vi "SCOnly.vi"() -> ()   [LabVIEW 2014]
uses:
  <vilib>/Instr/_visa.llb/VISA Configure Serial Port (Instr).vi
panel:
  in  "stop":bool
  in  "Abort SC":bool
  out "Si Abort Readout":string
  out "TL Abort readout":string
  in  "Si Test Steps":dbl format="%#_13g"
  out "Si Test String":string
  out "Si Test Readout":string
  in  "Si Test":bool=TRUE
  in  "TL Test Steps":dbl format="%#_13g"
  out "Tl Test String":string
  out "Tl Test Readout":string
  in  "TL Test":bool=TRUE
  in  "Si":T1(radio)=enum."Radio Selection 1"
  out "Si in Position? SC":bool=TRUE
  out "TL in Position? SC":bool=TRUE
  in  "Normal/Overide":bool=TRUE
  in  "TL":T2(radio)=enum."Radio Selection 1"
  out "Si Output":string
  out "Si Input":string
  out "TL Output":string
  out "TL Input":string
  in  "Pos5 Enable":bool=TRUE
  in  "Pos4 Enable":bool=TRUE
  in  "Pos3 Enable":bool=TRUE
  in  "Pos2 Enable":bool=TRUE
  in  "Pos1 Enable":bool=TRUE
  out "Si Position Readout":string
  out "TL Position Readout":string
  out "TL Position":i32
  out "TL Bar":i32(slide) scale=0.0..429000.0
  out "Si Position":i32
  out "Si Bar":i32(slide) scale=0.0..49001.0
  in  "SC On/Off":bool=TRUE
  in  "Si Speed Value":i32=2000
  in  "Si MID Value":i32=26000
  in  "Si IN Value":i32=49000
  in  "TL Speed Value":i32=4000
  in  "Pos5 Value":i32=429000
  in  "Pos4 Value":i32=339000
  in  "Pos3 Value":i32=249000
  in  "Pos2 Value":i32=163000
  in  "Pos1 Value":i32=71000
  out "Si \nSpeed":i32 min=0 format="%#.10f"
  out "Si MID":i32 min=0 format="%#.10f"
  out "Si IN":i32 min=0 format="%#.10f"
  out "TL \nSpeed":i32 min=0 format="%#.10f"
  out "Position5":i32 min=0 format="%#.10f"
  out "Position4":i32 min=0 format="%#.10f"
  out "Position3":i32 min=0 format="%#.10f"
  out "Position2":i32 min=0 format="%#.10f"
  out "Position1":i32 min=0 format="%#.10f"
  in  "TL/Si, Comm 29, C":refnum<visa-resource-name>="COM29"
  # "Faraday Cup"
  # "Si Home"
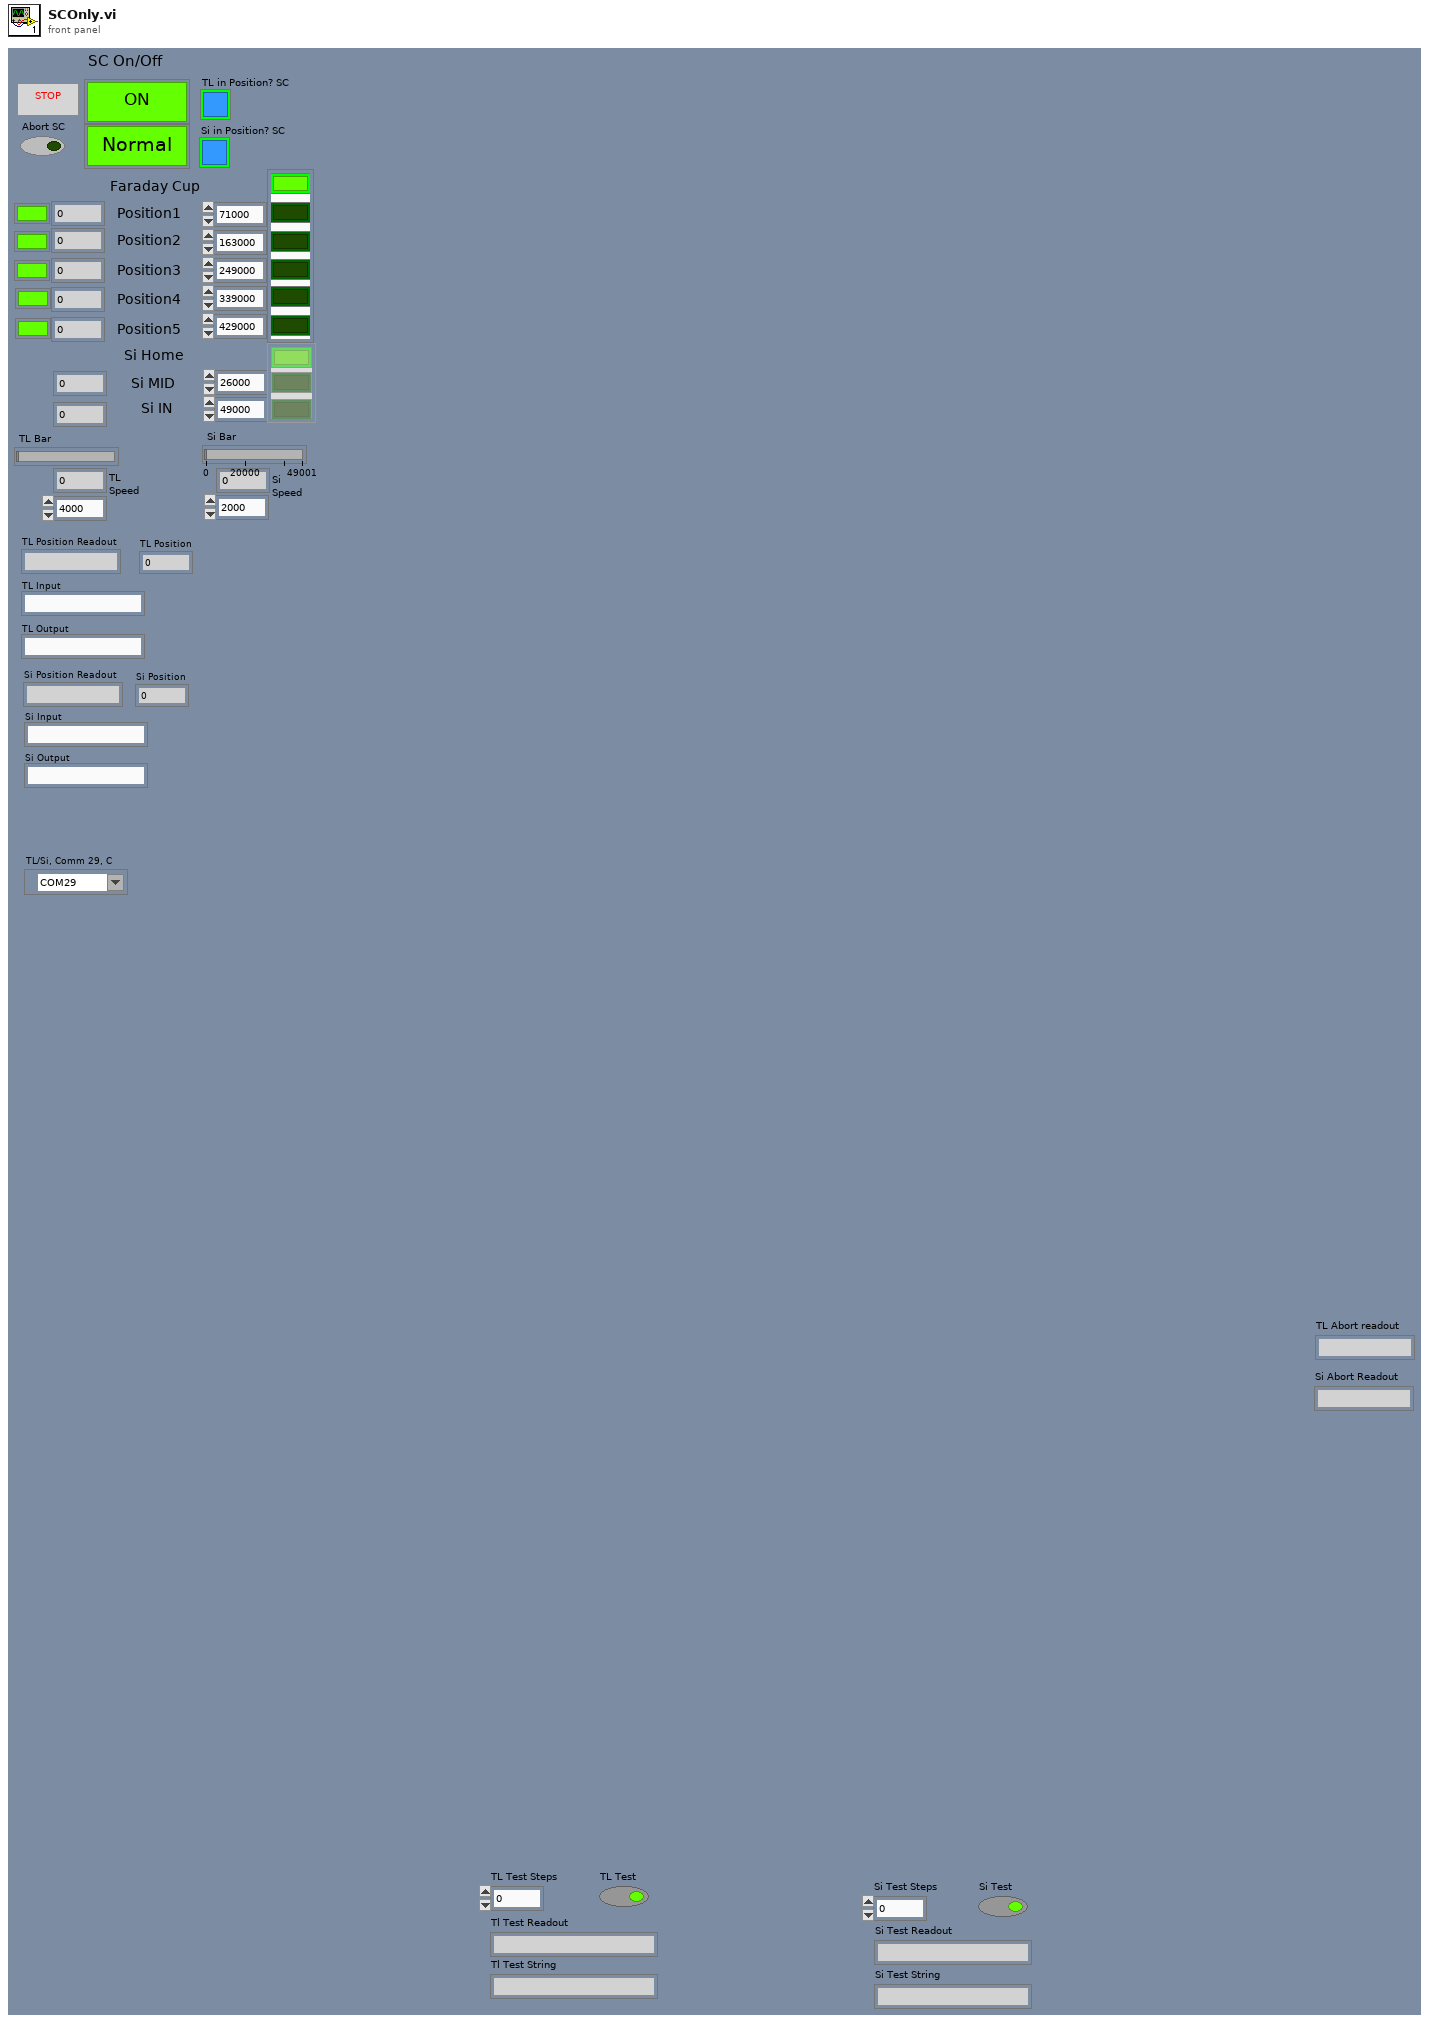
[diagram p1: front panel]
types:
  T1 = enum32{"No Selection", "Radio Selection 1", "Radio Selection 2", "Radio Selection 3"}
  T2 = enum32{"No Selection", "Radio Selection 1", "Radio Selection 2", "Radio Selection 3", "Radio Selection 4", "Radio Selection 5", "Radio Selection 6"}
  T3 = enum8{"Enabled", "Disabled", "Disabled and Grayed Out"}
  T4 = cluster{"read buffer":string, "Numeric":i32, "read buffer":string, "Numeric":i32, bool}
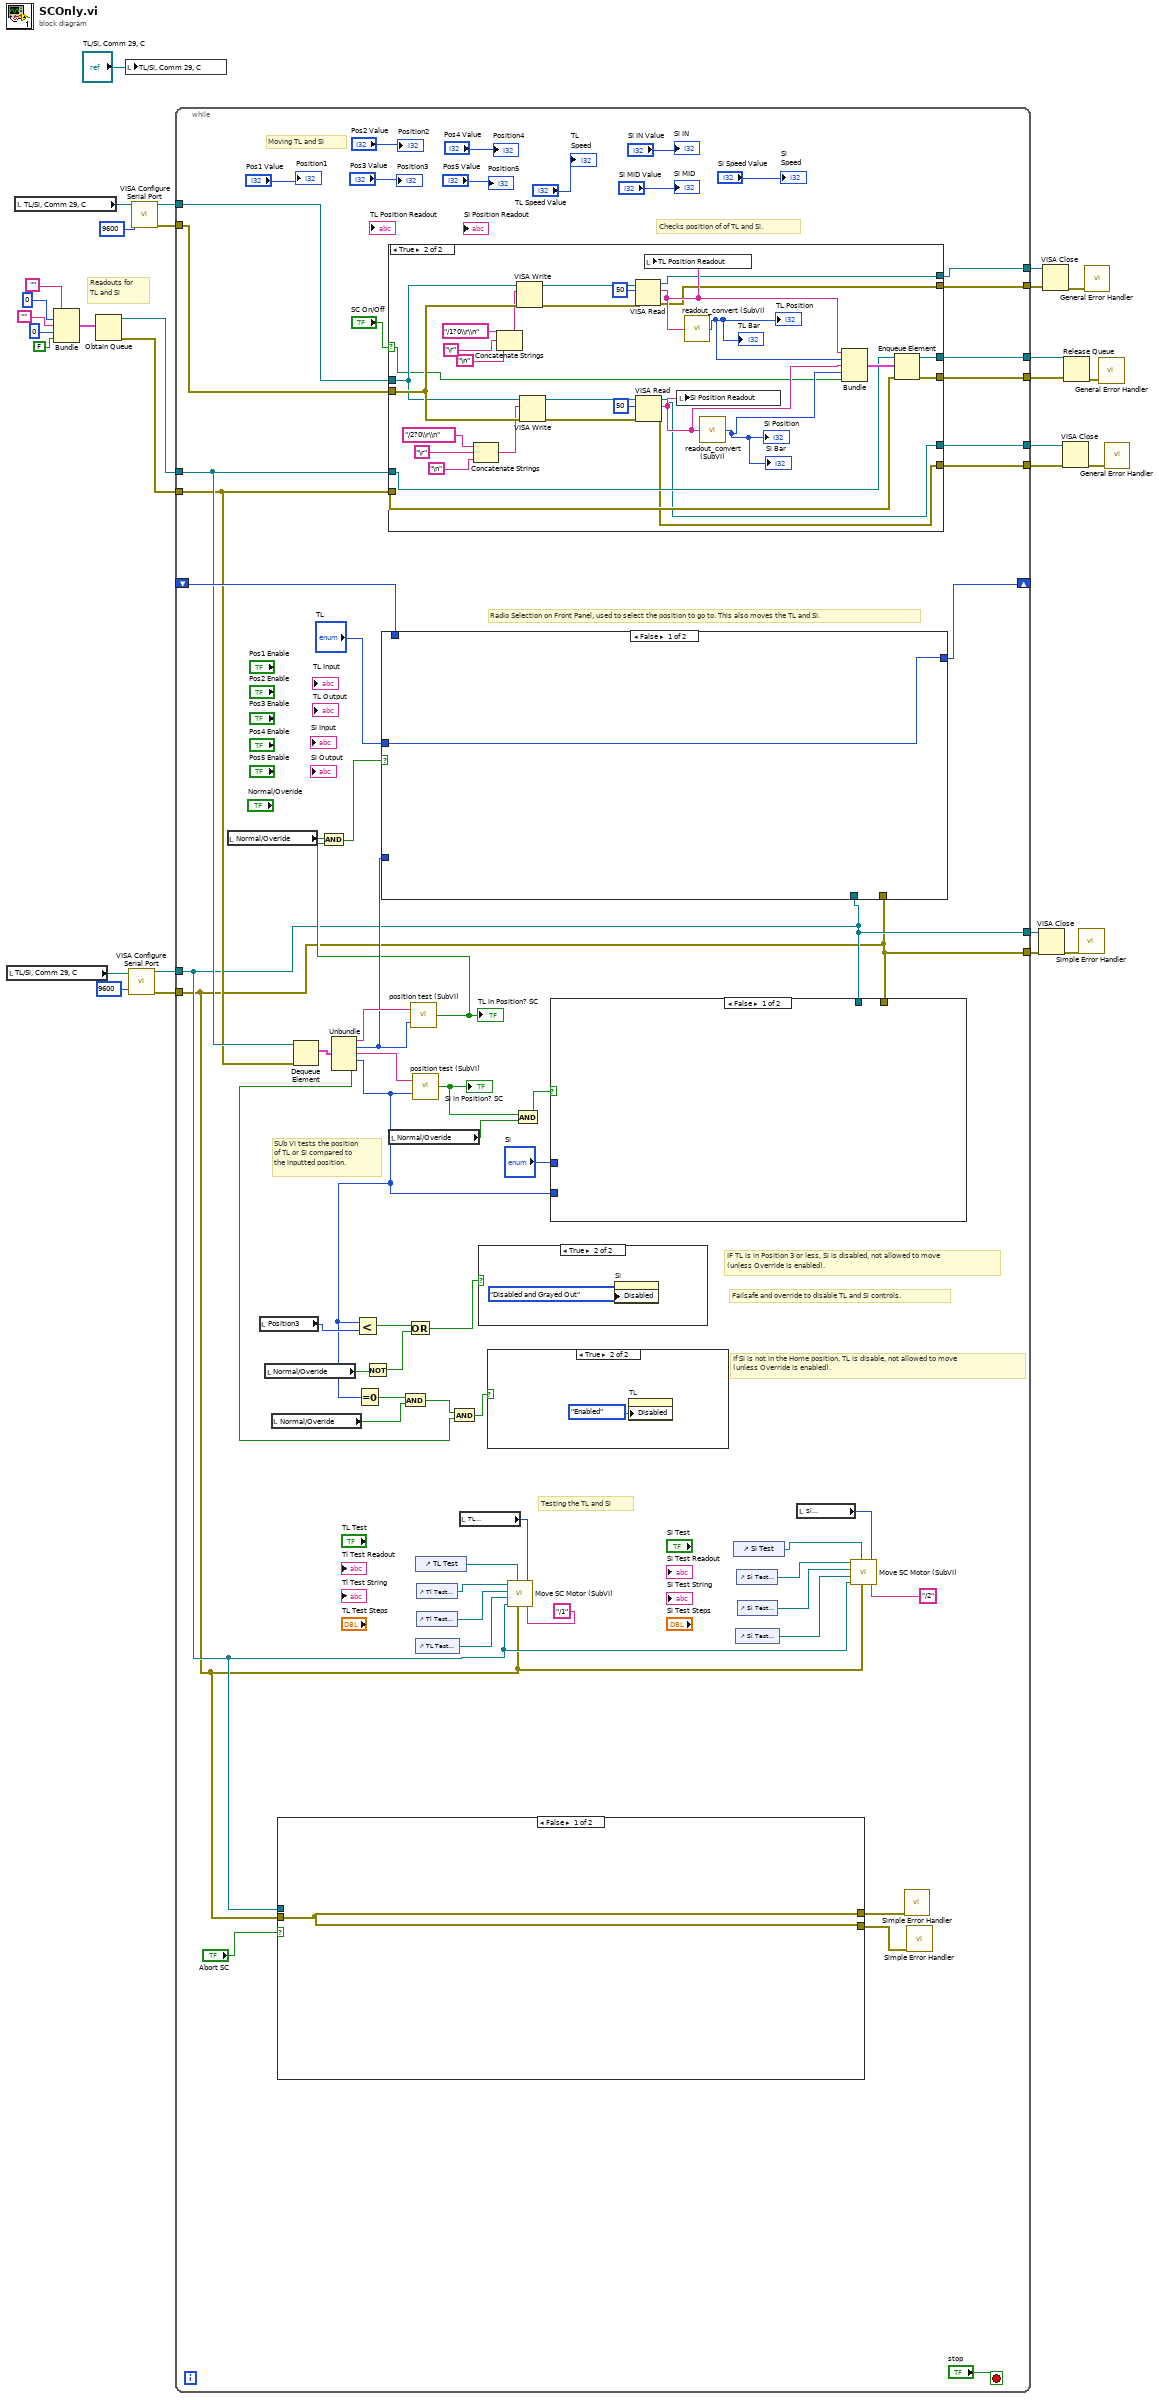
[diagram p0: block diagram]
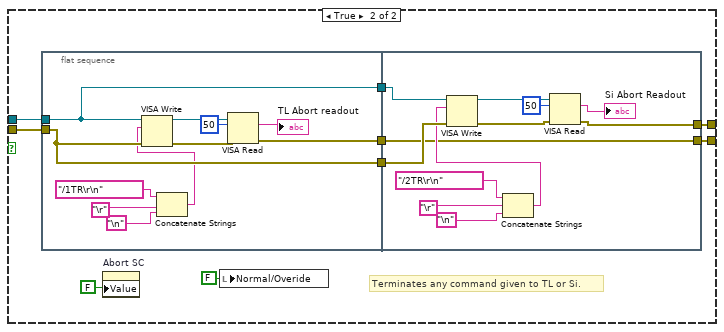
[diagram p2: hidden frame]
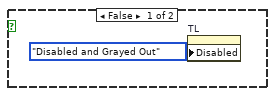
[diagram p3: hidden frame]
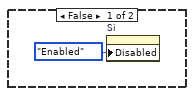
[diagram p4: hidden frame]
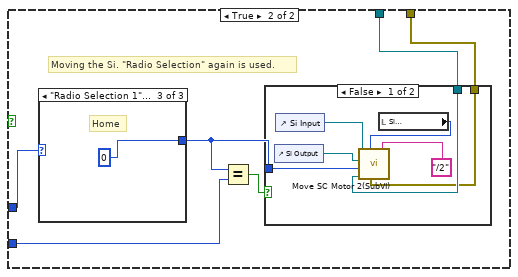
[diagram p5: hidden frame]
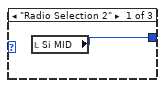
[diagram p7: hidden frame]
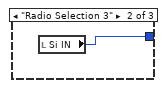
[diagram p8: hidden frame]
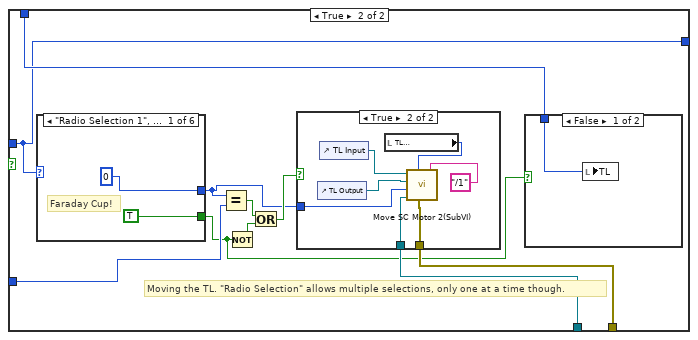
[diagram p9: hidden frame]
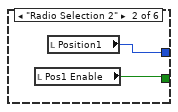
[diagram p12: hidden frame]
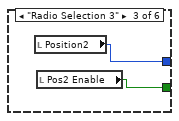
[diagram p13: hidden frame]
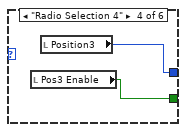
[diagram p14: hidden frame]
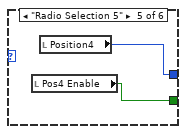
[diagram p15: hidden frame]
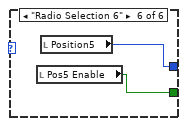
[diagram p16: hidden frame]
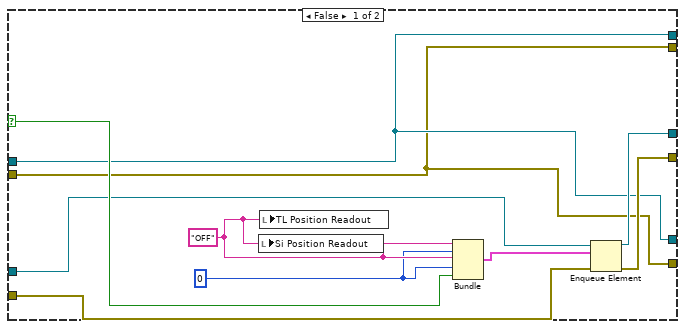
[diagram p17: hidden frame]
diagram:
  # "Readouts for \nTL and Si"
  n1 = local read "TL/Si, Comm 29, C"() -> (w11:refnum<visa-resource-name>)
  n2 = local read "TL/Si, Comm 29, C"() -> (w28:refnum<visa-resource-name>)
  n3 = Bundle("", 0, "", 0, FALSE) -> (w20:cluster{string, i32, string, i32, bool})  [unwired: 1 in]
  n4 = Obtain Queue(element data type=w20) -> (queue out=w19:refnum<queue>, error out=w18:errorcluster)  [unwired: 4 in, 1 out]
  n5 = local write "TL/Si, Comm 29, C"("TL/Si, Comm 29, C") -> ()
  n6 = call-poly "VISA Configure Serial Port"("VISA resource name"=w11, "baud rate (9600)"=u32 9600) -> ("VISA resource name out"=w10:refnum<visa-resource-name>, "error out"=w9:errorcluster)  [unwired: 12 in]
  n7 = call-poly "VISA Configure Serial Port"("VISA resource name"=w28, "baud rate (9600)"=u32 9600) -> ("VISA resource name out"=w27:refnum<visa-resource-name>, "error out"=w26:errorcluster)  [unwired: 12 in]
  n8 = while {
    tunnel: w27 -> [w81]
    tunnel: w26 -> [w82]
    tunnel: w19 -> [w70]
    tunnel: w18 -> [w69]
    tunnel: [w80] -> w15
    tunnel: [w79] -> w14
    tunnel: [w78] -> w13
    tunnel: [w77] -> w12
    shift-right: [w72] -> _
    shift-left: _ -> [w73]
    tunnel: w10 -> [w34]
    tunnel: w9 -> [w33]
    tunnel: [w34] -> w7
    tunnel: [w33] -> w6
    tunnel: [w31] -> w4
    tunnel: [w30] -> w3
    stop <- "stop" stop-if-true
    # "Testing the TL and Si"
    # "If Si is not in the Home position, TL is disable, not allowed to move\n(unless Override is enabled)."
    # "Failsafe and override to disable TL and Si controls."
    # "IF TL is in Position 3 or less, Si is disabled, not allowed to move\n(unless Override is enabled)."
    # "SUb Vi tests the position\nof TL or Si compared to\nthe inputted position."
    # "Radio Selection on Front Panel, used to select the position to go to. This also moves the TL and Si."
    # "Checks position of of TL and Si."
    # "Moving TL and Si"
    n9 = local read "Normal/Overide"() -> (w76:bool)
    n10 = local read "Position3"() -> (w60:i32)
    n11 = local read "Normal/Overide"() -> (w58:bool)
    n12 = local read "Normal/Overide"() -> (w54:bool)
    n13 = case shown="False" "Abort SC" {
      tunnel: w34 -> [_ w102]
      tunnel: w33 -> [w93 w100]
      tunnel: [w93 w97] -> w36
      tunnel: [w93 w96] -> w37
      frame False {
      }
      frame True {
        # "Terminates any command given to TL or Si."
        n14 = flat-sequence {
          tunnel: w102 -> [w112]
          tunnel: [w112] -> w101
          tunnel: w100 -> [w110]
          tunnel: [w110] -> w99
          tunnel: [w103] -> w98
          tunnel: w101 -> [w125]
          tunnel: w99 -> [w123]
          tunnel: w98 -> [w115]
          tunnel: [w115] -> w97
          tunnel: [w114] -> w96
          frame #0 {
            n15 = Concatenate Strings("/1TR\r\n", "\r", "\n") -> (w105:string)
            n16 = VISA Write(VISA resource name=w112, write buffer=w105, error in (no error)=w110) -> (VISA resource name out=w113:refnum<visa-resource-name>, error out=w111:errorcluster)  [unwired: 1 out]
            n17 = VISA Read(VISA resource name=w113, byte count=u32 50, error in (no error)=w111) -> (read buffer=→"TL Abort readout":string, error out=w103:errorcluster)  [unwired: 2 out]
          }
          frame #1 {
            n18 = Concatenate Strings("/2TR\r\n", "\r", "\n") -> (w117:string)
            n19 = VISA Write(VISA resource name=w125, write buffer=w117, error in (no error)=w123) -> (VISA resource name out=w124:refnum<visa-resource-name>, error out=w122:errorcluster)  [unwired: 1 out]
            n20 = VISA Read(VISA resource name=w124, byte count=u32 50, error in (no error)=w122) -> (read buffer=→"Si Abort Readout":string, error out=w114:errorcluster)  [unwired: 2 out]
          }
        }
        n21 = property on="Abort SC" class="Bool (strict)"("Value"=FALSE ("Abort SC")) -> ()  [unwired: 2 in, 2 out]
        n22 = local write "Normal/Overide"(FALSE ("Normal/Overide")) -> ()
      }
    }
    n23 = Dequeue Element(queue=w70, error in (no error)=w69) -> (element=w71:cluster{string, i32, string, i32, bool})  [unwired: 1 in, 3 out]
    n24 = Unbundle(w71) -> (w68:string, w66:i32, w67:string, w56:i32, w52:bool)
    n25 = Less?(x=w56, y=w60) -> (x < y?=w59:bool)
    n26 = Equal To 0?(x=w56) -> (x = 0?=w55:bool)
    n27 = Not(x=w58) -> (.not. x?=w57:bool)
    n28 = case shown="True" "SC On/Off" {
      selector: "SC On/Off" -> [w184 w193]
      tunnel: w81 -> [w178 w212]
      tunnel: w82 -> [w177 w216]
      tunnel: w70 -> [w182 w201]
      tunnel: w69 -> [w181 w200]
      tunnel: [w180 w199] -> w78
      tunnel: [w179 w198] -> w77
      tunnel: [w178 w196] -> w80
      tunnel: [w177 w197] -> w79
      tunnel: [w178 w195] -> w31
      tunnel: [w177 w194] -> w30
      frame False {
        w185 = 0
        w186 = "OFF"
        n29 = local write "Si Position Readout"(w186) -> ()
        n30 = local write "TL Position Readout"(w186) -> ()
        n31 = Bundle(w186, w185, w186, w185, w184) -> (w183:cluster{string, i32, string, i32, bool})  [unwired: 1 in]
        n32 = Enqueue Element(queue=w182, element=w183, error in (no error)=w181) -> (queue out=w180:refnum<queue>, error out=w179:errorcluster)  [unwired: 1 in, 1 out]
      }
      frame True {
        n33 = Concatenate Strings("/2?0\\r\\n", "\r", "\n") -> (w205:string)
        n34 = Concatenate Strings("/1?0\\r\\n", "\r", "\n") -> (w211:string)
        n35 = VISA Write(VISA resource name=w212, write buffer=w211, error in (no error)=w216) -> (VISA resource name out=w192:refnum<visa-resource-name>, error out=w191:errorcluster)  [unwired: 1 out]
        n36 = VISA Write(VISA resource name=w212, write buffer=w205, error in (no error)=w216) -> (VISA resource name out=w189:refnum<visa-resource-name>, error out=w188:errorcluster)  [unwired: 1 out]
        n37 = VISA Read(VISA resource name=w192, byte count=u32 50, error in (no error)=w191) -> (VISA resource name out=w196:refnum<visa-resource-name>, read buffer=w210:string, error out=w197:errorcluster)  [unwired: 1 out]
        n38 = VISA Read(VISA resource name=w189, byte count=u32 50, error in (no error)=w188) -> (VISA resource name out=w195:refnum<visa-resource-name>, read buffer=w204:string, error out=w194:errorcluster)  [unwired: 1 out]
        n39 = local write "TL Position Readout"(w210) -> ()
        n40 = local write "Si Position Readout"(w204) -> ()
        n41 = call "readout_convert (SubVI).vi"("read buffer"=w210) -> ("Numeric"=w209:i32)
        "TL Position" <- w209
        "TL Bar" <- w209
        n42 = call "readout_convert (SubVI).vi"("read buffer"=w204) -> ("Numeric"=w203:i32)
        "Si Position" <- w203
        "Si Bar" <- w203
        n43 = Bundle("read buffer"=w210, "Numeric"=w209, "read buffer"=w204, "Numeric"=w203, w193) -> (w202:T4)  [unwired: 1 in]
        n44 = Enqueue Element(queue=w201, element=w202, error in (no error)=w200) -> (queue out=w199:refnum<queue>, error out=w198:errorcluster)  [unwired: 1 in, 1 out]
      }
    }
    n45 = local read "Normal/Overide"() -> (w61:bool)
    n46 = And(x=w55, y=w54) -> (x .and. y?=w53:bool)
    n47 = Or(x=w59, y=w57) -> (x .or. y?=w51:bool)
    n48 = call "position test (SubVI).vi"("Numeric"=w66, "String"=w68) -> ("Boolean"=w65:bool)
    "TL in Position? SC" <- w65
    n49 = And(x=w76, y=w65) -> (x .and. y?=w75:bool)
    n50 = case shown="False" w75 {
      tunnel: "TL" -> [w146 w152]
      tunnel: w73 -> [_ w153]
      tunnel: [w146 w152] -> w72
      tunnel: w66 -> [_ w151]
      tunnel: w34 -> [_ w149]
      tunnel: w33 -> [_ w148]
      frame False {
      }
      frame True {
        # "Moving the TL. \"Radio Selection\" allows multiple selections, only one at a time though."
        n51 = case shown="\"Radio Selection 1\", Default" w152 {
          tunnel: [0 w168 w170 w172 w174 w176] -> w150
          tunnel: [TRUE w167 w169 w171 w173 w175] -> w147
          frame "Radio Selection 1", Default {
            # "Faraday Cup!"
          }
          frame "Radio Selection 2" {
            n52 = local read "Pos1 Enable"() -> (w167:bool)
            n53 = local read "Position1"() -> (w168:i32)
          }
          frame "Radio Selection 3" {
            n54 = local read "Position2"() -> (w170:i32)
            n55 = local read "Pos2 Enable"() -> (w169:bool)
          }
          frame "Radio Selection 4" {
            n56 = local read "Pos3 Enable"() -> (w171:bool)
            n57 = local read "Position3"() -> (w172:i32)
          }
          frame "Radio Selection 5" {
            n58 = local read "Pos4 Enable"() -> (w173:bool)
            n59 = local read "Position4"() -> (w174:i32)
          }
          frame "Radio Selection 6" {
            n60 = local read "Pos5 Enable"() -> (w175:bool)
            n61 = local read "Position5"() -> (w176:i32)
          }
        }
        n62 = Equal?(x=w150, y=w151) -> (x = y?=w154:bool)
        n63 = Not(x=w147) -> (.not. x?=w155:bool)
        n64 = Or(x=w154, y=w155) -> (x .or. y?=w156:bool)
        n65 = case shown="True" w156 {
          tunnel: w150 -> [_ w160]
          tunnel: w149 -> [_ w159]
          tunnel: w148 -> [_ w158]
          frame False {
          }
          frame True {
            n66 = control-ref of="TL Output"() -> (w163:refnum<vi>)
            n67 = control-ref of="TL Input"() -> (w164:refnum<vi>)
            n68 = local read "TL \nSpeed"() -> (w162:i32)
            n69 = call "Move SC Motor 2(SubVI).vi"("String"="/1", "error out"=w158, "Speed"=w162, "VISA resource name out"=w159, "Position"=w160, "Output"=w163, "Input"=w164) -> ()
          }
        }
        n70 = case shown="False" w147 {
          tunnel: w153 -> [w157 _]
          frame False {
            n71 = local write "TL"(w157) -> ()
          }
          frame True {
          }
        }
      }
    }
    n72 = call "position test (SubVI).vi"("Numeric"=w56, "String"=w67) -> ("Boolean"=w62:bool)
    "Si in Position? SC" <- w62
    n73 = control-ref of="TL Test Steps"() -> (w45:refnum<vi>)
    n74 = control-ref of="TL Test"() -> (w48:refnum<vi>)
    n75 = control-ref of="Tl Test Readout"() -> (w47:refnum<vi>)
    n76 = control-ref of="Tl Test String"() -> (w46:refnum<vi>)
    n77 = And(x=w53, y=w52) -> (x .and. y?=w50:bool)
    n78 = local read "TL \nSpeed"() -> (w49:i32)
    n79 = case shown="True" w51 {
      frame False {
        n80 = property on="Si" class="RadioBtnsControl (strict)"("Disabled"=T3."Enabled") -> ()  [unwired: 2 in, 2 out]
      }
      frame True {
        n81 = property on="Si" class="RadioBtnsControl (strict)"("Disabled"=T3."Disabled and Grayed Out") -> ()  [unwired: 2 in, 2 out]
      }
    }
    n82 = case shown="True" w50 {
      frame False {
        n83 = property on="TL" class="RadioBtnsControl (strict)"("Disabled"=T3."Disabled and Grayed Out") -> ()  [unwired: 2 in, 2 out]
      }
      frame True {
        n84 = property on="TL" class="RadioBtnsControl (strict)"("Disabled"=T3."Enabled") -> ()  [unwired: 2 in, 2 out]
      }
    }
    n85 = call "Move SC Motor (SubVI).vi"("String"="/1", "Speed"=w49, "error out"=w33, "Button"=w48, "VISA resource name out"=w34, "Steps"=w45, "Output"=w46, "Input"=w47) -> ()
    n86 = And(x=w62, y=w61) -> (x .and. y?=w64:bool)
    n87 = case shown="False" w64 {
      tunnel: "Si" -> [_ w135]
      tunnel: w56 -> [_ w134]
      tunnel: w34 -> [_ w131]
      tunnel: w33 -> [_ w130]
      frame False {
      }
      frame True {
        # "Moving the Si. \"Radio Selection\" again is used."
        n88 = case shown="\"Radio Selection 1\", Default" w135 {
          tunnel: [w143 w144 0] -> w132
          frame "Radio Selection 2" {
            n89 = local read "Si MID"() -> (w143:i32)
          }
          frame "Radio Selection 3" {
            n90 = local read "Si IN"() -> (w144:i32)
          }
          frame "Radio Selection 1", Default {
            # "Home"
          }
        }
        n91 = Equal?(x=w132, y=w134) -> (x = y?=w133:bool)
        n92 = case shown="False" w133 {
          tunnel: w132 -> [w142 _]
          tunnel: w131 -> [w139 _]
          tunnel: w130 -> [w138 _]
          frame False {
            n93 = control-ref of="Si Output"() -> (w136:refnum<vi>)
            n94 = control-ref of="Si Input"() -> (w137:refnum<vi>)
            n95 = local read "Si \nSpeed"() -> (w141:i32)
            n96 = call "Move SC Motor 2(SubVI).vi"("String"="/2", "error out"=w138, "Speed"=w141, "VISA resource name out"=w139, "Position"=w142, "Output"=w136, "Input"=w137) -> ()
          }
          frame True {
          }
        }
      }
    }
    n97 = control-ref of="Si Test"() -> (w42:refnum<vi>)
    n98 = control-ref of="Si Test Steps"() -> (w39:refnum<vi>)
    n99 = control-ref of="Si Test Readout"() -> (w41:refnum<vi>)
    n100 = control-ref of="Si Test String"() -> (w40:refnum<vi>)
    n101 = local read "Si \nSpeed"() -> (w43:i32)
    n102 = call "Move SC Motor (SubVI).vi"("String"="/2", "Speed"=w43, "error out"=w33, "Button"=w42, "VISA resource name out"=w34, "Steps"=w39, "Output"=w40, "Input"=w41) -> ()
    n103 = call <vilib>:"Simple Error Handler.vi"("error in (no error)"=w37) -> ()  [unwired: 4 in, 5 out]
    n104 = call <vilib>:"Simple Error Handler.vi"("error in (no error)"=w36) -> ()  [unwired: 4 in, 5 out]
    "Position1" <- "Pos1 Value"
    "Position2" <- "Pos2 Value"
    "Position3" <- "Pos3 Value"
    "Position4" <- "Pos4 Value"
    "Position5" <- "Pos5 Value"
    "TL \nSpeed" <- "TL Speed Value"
    "Si IN" <- "Si IN Value"
    "Si MID" <- "Si MID Value"
    "Si \nSpeed" <- "Si Speed Value"
  }
  n105 = VISA Close(VISA resource name=w7, error in (no error)=w6) -> (error out=w8:errorcluster)
  n106 = VISA Close(VISA resource name=w15, error in (no error)=w14) -> (error out=w17:errorcluster)
  n107 = VISA Close(VISA resource name=w4, error in (no error)=w3) -> (error out=w5:errorcluster)
  n108 = Release Queue(queue=w13, error in (no error)=w12) -> (error out=w16:errorcluster)  [unwired: 1 in, 2 out]
  n109 = call <vilib>:"Simple Error Handler.vi"("error in (no error)"=w8) -> ()  [unwired: 4 in, 5 out]
  n110 = call <vilib>:"General Error Handler.vi"("error in (no error)"=w17) -> ()  [unwired: 10 in, 5 out]
  n111 = call <vilib>:"General Error Handler.vi"("error in (no error)"=w16) -> ()  [unwired: 10 in, 5 out]
  n112 = call <vilib>:"General Error Handler.vi"("error in (no error)"=w5) -> ()  [unwired: 10 in, 5 out]
